vi "Audio Filtering (Time Domain).vi"(0 "waveforms":waveform(dbl)[](array[waveform]), 1 "filter settings":T1={"weighting filter"=20, "highpass filter"=enum."AC", "lowpass filter "=enum."AES17 20kHz"} {"weighting filter" items=["Linear", "A-weighting", "B-weighting", "C-weighting"]}, 3 "error in":errorcluster) -> (7 "time domain":waveform(dbl)[](array[waveform]), 10 "error out":errorcluster)   [LabVIEW 2021]
uses:
  controls/audio filter settings.ctl
  audio highpass filter type.ctl
  audio lowpass filter type.ctl
  <vilib>/addons/_NISVFA/_Shared subVIs/Controls/svc_Window.ctl
  <vilib>/addons/Sound and Vibration/svt_Level/SVL AC & DC Level (Time) (N Ch).vi
  <vilib>/addons/Sound and Vibration/svt_Level/SVL AC & DC Level (Time) (1 Ch).vi
  <vilib>/addons/_NISVFA/_Shared subVIs/Common/svc_Get SV Channel Info.vi
  <vilib>/Analysis/baseanly.llb/Mean.vi
  <vilib>/Analysis/baseanly.llb/Mean (DBL).vi
  <vilib>/addons/_NISVFA/_Shared subVIs/Windowing/svfa_Scaled Time Domain Window (Array).vi
  <vilib>/addons/_NISVFA/_Shared subVIs/Common/svc_Unit Label to Engineering Units.vi
  <vilib>/addons/_NISVFA/_Shared subVIs/Common/svc_Engineering Units to Unit Label.vi
  <vilib>/addons/_NISVFA/_Spectrum Processing/subVIs/svfa_Spectrum Info Window to windowTd Type Def.vi
  <vilib>/Analysis/4window.llb/Force Window.vi
  <vilib>/Analysis/4window.llb/Force Window (DBL).vi
  <vilib>/Analysis/4window.llb/Exponential Window.vi
  <vilib>/Analysis/4window.llb/Exponential Window (DBL).vi
  <vilib>/addons/_NISVFA/_Shared subVIs/Common/svc_Get Window Info.vi
  <vilib>/Analysis/0measdsp.llb/Scaled Time Domain Window.vi
  <vilib>/Analysis/0measdsp.llb/Scaled Time Domain Window (DBL).vi
  <vilib>/Utility/error.llb/Error Cluster From Error Code.vi
  <vilib>/Analysis/baseanly.llb/Std Deviation and Variance.vi
  <vilib>/addons/_NISVFA/_Shared subVIs/Common/svc_Caller VI Returned in Error Source.vi
  <vilib>/addons/Sound and Vibration/svt_Weighting/SVT Audio Filter (N Ch).vi
  <vilib>/addons/Sound and Vibration/svt_Weighting/SVT Weighting Filter (N Ch).vi
  <vilib>/addons/Sound and Vibration/svt_Weighting/SoundVib_ABCWeighting.lvlib
  <vilib>/addons/Sound and Vibration/svt_Weighting/SoundVib_AudioFilter.lvlib
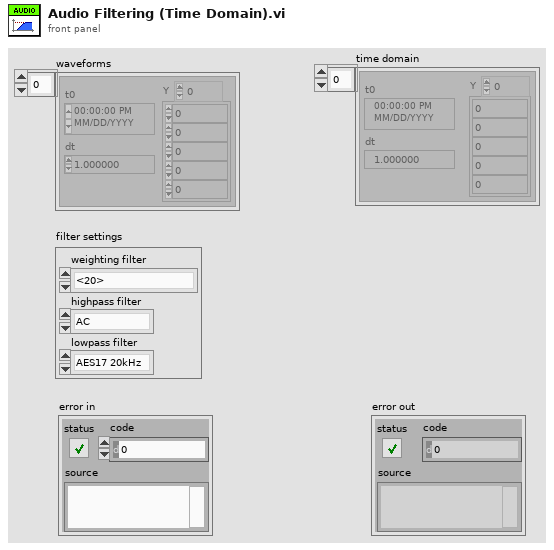
[diagram p1: front panel]
types:
  T1 = typedef "audio filter settings.ctl" = cluster{"weighting filter":u16, "highpass filter":T2, "lowpass filter ":T3}
  T2 = typedef "audio highpass filter type.ctl" = enum32{"DC", "AC"}
  T3 = typedef "audio lowpass filter type.ctl" = enum32{"No filter", "AES17 20kHz", "AES17 40kHz"}
  T4 = typedef "svc_Window.ctl" = u32
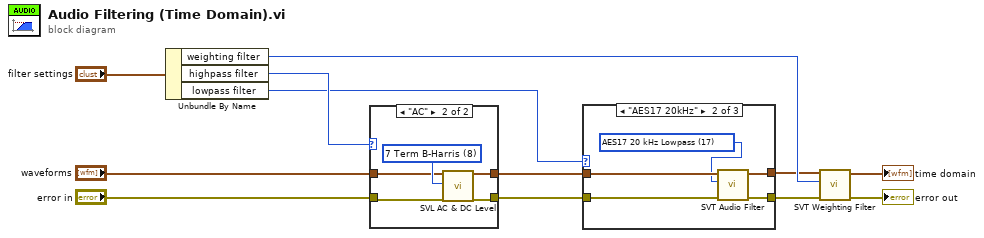
[diagram p0: block diagram]
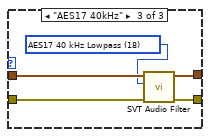
[diagram p3: hidden frame]
diagram:
  n1 = Unbundle By Name("filter settings") -> ("weighting filter"=w11:u16, "highpass filter"=w10:T2, "lowpass filter"=w7:T3)
  n2 = case shown="\"AC\"" w10 {
    tunnel: "error in" -> [w13 w17]
    tunnel: "waveforms" -> [w14 w18]
    tunnel: [w14 w16] -> w6
    tunnel: [w13 w15] -> w5
    frame "DC", Default {
    }
    frame "AC" {
      w19 = T4 8 items=["None"=0, "Hanning"=1, "Hamming"=2, "Blackman-Harris"=3, "Exact Blackman"=4, "Blackman"=5, "Flat Top"=6, "4 Term B-Harris "=7, "7 Term B-Harris"=8, "Low Sidelobe"=9, "Force"=64, "Exponential"=65, "Blackman Nuttall"=11, "Triangle"=30, "Bartlett-Hanning"=31, "Bohman"=32, "Parzen"=33, "Welch"=34, "Kaiser"=60, "Dolph-Chebyshev"=61, "Gaussian"=62] ("window")
      n3 = call-poly <vilib>:"SVL AC & DC Level.vi"("scaled signals in [EU]"=w18, "window"=w19, "error in (no error)"=w17) -> ("AC signals [EU]"=w16:waveform(dbl)[], "error out"=w15:errorcluster)  [unwired: 11 in, 4 out]
    }
  }
  n4 = case shown="\"AES17 20kHz\"" w7 {
    tunnel: w6 -> [w21 w26 w31]
    tunnel: w5 -> [w20 w25 w30]
    tunnel: [w21 w24 w29] -> w4
    tunnel: [w20 w23 w28] -> w3
    frame "No filter", Default {
    }
    frame "AES17 20kHz" {
      w22 = u16 17 items=["Linear"=0, "AES17 20 kHz Lowpass"=17, "AES17 40 kHz Lowpass"=18, "AES17 20 kHz Highpass"=19, "AES17 40 kHz Highpass"=20] ("filter type")
      n5 = call-poly <vilib>:"SVT Audio Filter.vi"("error in (no error)"=w25, "filter type"=w22, "scaled signals [EU]"=w26) -> ("error out"=w23:errorcluster, "filtered signals [EU]"=w24:waveform(dbl)[])  [unwired: 5 in, 2 out]
    }
    frame "AES17 40kHz" {
      w27 = u16 18 items=["Linear"=0, "AES17 20 kHz Lowpass"=17, "AES17 40 kHz Lowpass"=18, "AES17 20 kHz Highpass"=19, "AES17 40 kHz Highpass"=20] ("filter type")
      n6 = call-poly <vilib>:"SVT Audio Filter.vi"("error in (no error)"=w30, "filter type"=w27, "scaled signals [EU]"=w31) -> ("error out"=w28:errorcluster, "filtered signals [EU]"=w29:waveform(dbl)[])  [unwired: 5 in, 2 out]
    }
  }
  n7 = call-poly <vilib>:"SVT Weighting Filter.vi"("error in (no error)"=w3, "weighting"=w11, "scaled signals [EU]"=w4) -> ("error out"=→"error out":errorcluster, "weighted signals [EU]"=→"time domain":waveform(dbl)[])  [unwired: 6 in]
